vi "Write channel info.vi"(8 "error in (no error)":errorcluster, 10 "channel info":T1, 11 "DSFChannel in":refnum<class "DSFChannel.lvclass">) -> (0 "error out":errorcluster, 3 "DSFChannel out":refnum<class "DSFChannel.lvclass">)   [LabVIEW 2017, in "DSFChannel.lvclass"]
uses:
  DSFChannel.lvclass
  Controls/dsf configuration file/1.0.0/dsf channel.ctl
  DSFChannel.lvclass/DSFChannel.ctl
  Controls/dsf configuration file/1.0.0/dsf configuration file v1.0.0.lvlib
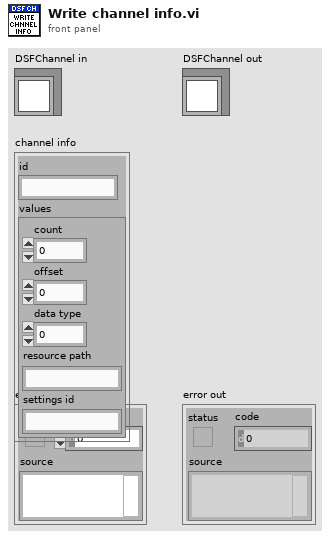
[diagram p1: front panel]
types:
  T1 = typedef "dsf configuration file v1.0.0.lvlib/dsf channel.ctl" = cluster{"id":string, "values":cluster{"count":i32, "offset":i32, "data type":i32, "resource path":string, "settings id":string}}
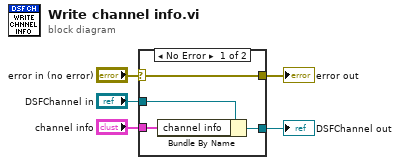
[diagram p0: block diagram]
diagram:
  n1 = case shown="No Error" "error in (no error)" {
    selector: "error in (no error)" -> [w9 w10]
    tunnel: [w9 w10] -> w4
    tunnel: [w7 w11] -> w2
    tunnel: "DSFChannel in" -> [w8 w11]
    tunnel: "channel info" -> [w6 _]
    frame No Error {
      n2 = Bundle By Name(cluster=w8, "channel info"=w6) -> (w7:refnum<class "DSFChannel.lvclass">)
    }
    frame Error {
    }
  }
  "error out" <- w4
  "DSFChannel out" <- w2
